vi "General Data Query.vi"(8 "error in (no error)":errorcluster, 10 "Data Enum":T1, 11 "Sensor General Class in":refnum<class "Sensor General Class.lvclass">) -> (0 "error out":errorcluster, 3 "Sensor General Class out":refnum<class "Sensor General Class.lvclass">)   [LabVIEW 2020, in "Sensor General Class.lvclass"]
uses:
  Sensor General Class.lvclass
  Data Enum.ctl
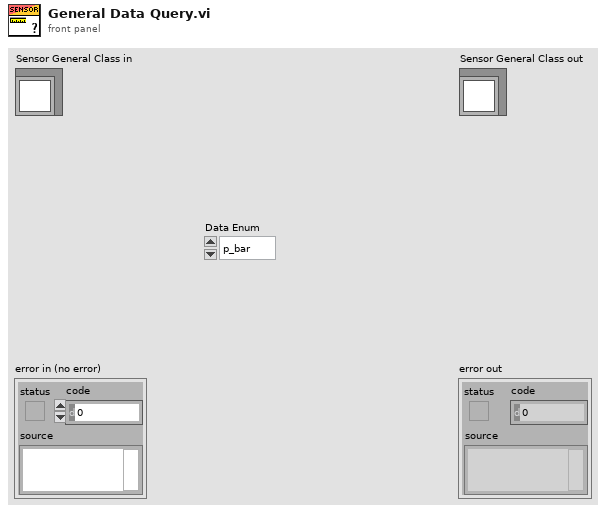
[diagram p1: front panel]
types:
  T1 = typedef "Sensor General Class.lvclass/Data Enum.ctl" = enum16{"p_bar", "p_MPa", "p_Pa", "p_kPa", "p_psi", "p_H/cm^2", "t_C", "t_K", "t_F", "rho_g/l", "rho_kg/m^3", "p20_bar", "related p20_bar", "p20_MPa", "related p20_MPa", "Tf_SF6", "Td_sf6", "tank Tf_SF6", "tank Td_SF6", "Tf_N2", "Td_N2", "tank Tf_N2", "tank Td_N2", "ppm_v SF6", "ppm_w SF6", "ppm_v N2", "ppm_w N2", "rH"}
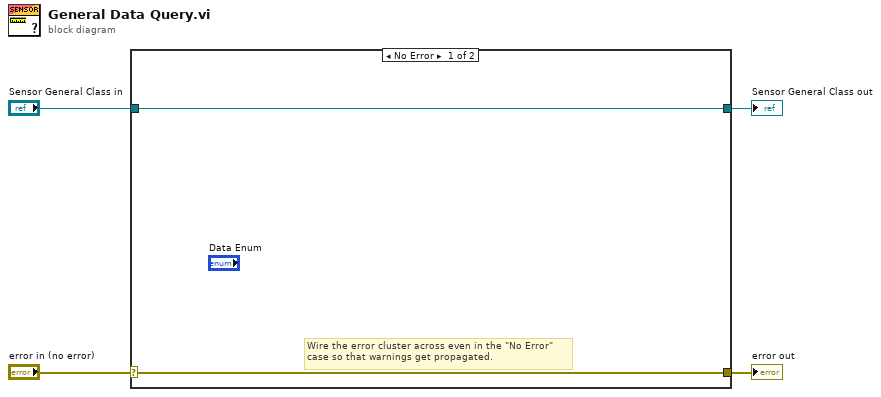
[diagram p0: block diagram]
diagram:
  n1 = case shown="No Error" "error in (no error)" {
    selector: "error in (no error)" -> [w5 w8]
    tunnel: [w5 w8] -> w3
    tunnel: [w6 w7] -> w1
    tunnel: "Sensor General Class in" -> [w6 w7]
    frame No Error {
      # "Wire the error cluster across even in the \"No Error\"\ncase so that warnings get propagated."
    }
    frame Error {
    }
  }
  "error out" <- w3
  "Sensor General Class out" <- w1
